vi "LIFO_INT_SVI.vi"(7 "OP":T1=enum."Push", 8 "error in (no error)":errorcluster, 10 "IN":i32, 11 "Array IN":i32[](array[numeric])) -> (0 "error out":errorcluster, 1 "Size":i32, 2 "Elem":i32, 3 "Array":i32[](array[numeric]))   [LabVIEW 2015]
uses:
  LIFO.ctl
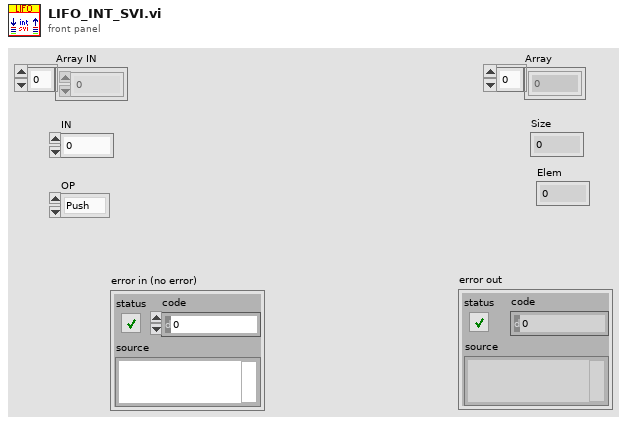
[diagram p1: front panel]
types:
  T1 = typedef "LIFO.ctl" = enum16{"INIT", "Push", "Pop", "Query", "BPush"}
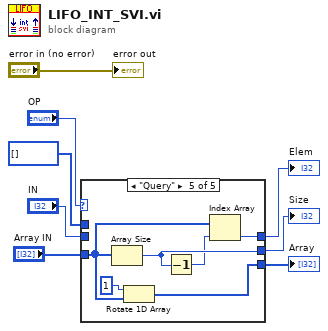
[diagram p0: block diagram]
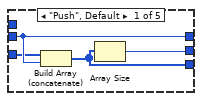
[diagram p2: hidden frame]
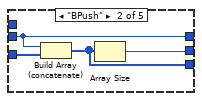
[diagram p3: hidden frame]
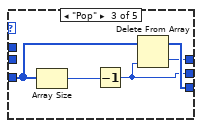
[diagram p4: hidden frame]
diagram:
  n1 = case shown="\"Query\"" "OP" {
    tunnel: "Array IN" -> [w11 w16 w21 _ w25]
    tunnel: "IN" -> [w12 w13 _ _ _]
    tunnel: [w10 w15 w20 w22 w24] -> w3
    tunnel: [w12 w13 w19 _ w26] -> w6
    tunnel: i32[] [] -> [_ _ _ w22 _]
    tunnel: [w9 w14 w17 _ w28] -> w4
    frame "Push", Default {
      n2 = Build Array (concatenate)(w11, w12) -> (w10:i32[])
      n3 = Array Size(array=w10) -> (size(s)=w9:i32)
    }
    frame "BPush" {
      n4 = Build Array (concatenate)(w13, w16) -> (w15:i32[])
      n5 = Array Size(array=w15) -> (size(s)=w14:i32)
    }
    frame "Pop" {
      n6 = Array Size(array=w21) -> (size(s)=w18:i32)
      n7 = Decrement(x=w18) -> (x-1=w17:i32)
      n8 = Delete From Array(array=w21, index=w17) -> (deleted portion=w19:i32, array with subset deleted=w20:i32[])  [unwired: 1 in]
    }
    frame "INIT" {
    }
    frame "Query" {
      n9 = Array Size(array=w25) -> (size(s)=w28:i32)
      n10 = Rotate 1D Array(1:w25, 2:1 ("n")) -> (0:w24:i32[])
      n11 = Decrement(x=w28) -> (x-1=w27:i32)
      n12 = Index Array(array=w25, index=w27) -> (element=w26:i32)
    }
  }
  "Elem" <- w6
  "Size" <- w4
  "Array" <- w3
  "error out" <- "error in (no error)"
